vi "Setup measurement.vi"(8 "error in (no error)":errorcluster, 11 "VISA resource name":refnum<visa-resource-name>) -> (0 "error out":errorcluster, 3 "VISA resource name out":refnum<visa-resource-name>)   [LabVIEW 2021]
uses:
  <instrlib>/Keithley 2450/Keithley 2450.lvlib
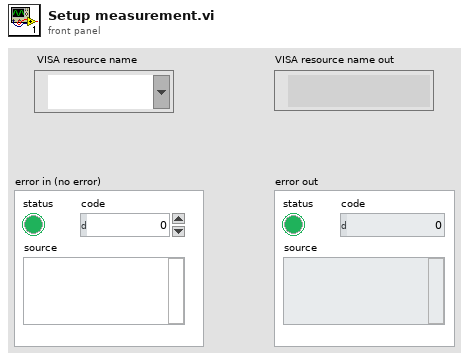
[diagram p1: front panel]
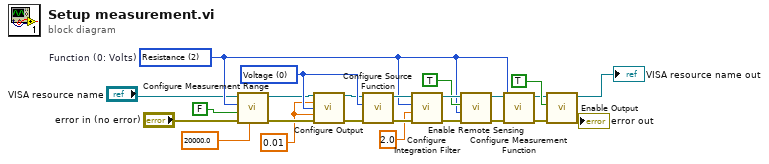
[diagram p0: block diagram]
diagram:
  w24 = u16 0 items=["Voltage", "Current"] ("Source Mode  (0: Voltage)")
  w6 = 0.01 ("Output Level (0)")
  w5 = u16 2 items=["Volts", "Current", "Resistance"]  # Function (0: Volts)
  n1 = call <instrlib>:"Configure Measurement Range.vi"("Manual Range (1.0)"=20000.0 ("Measurement Speed (1 PLC)"), "error in (no error)"="error in (no error)", "Enable Auto Range (T:Enable)"=FALSE, "Function (0: Volts)"=w5, "VISA resource name"="VISA resource name") -> ("error out"=w19:errorcluster, "VISA resource name out"=w20:refnum<visa-resource-name>)  [unwired: 5 in]
  n2 = call <instrlib>:"Configure Output.vi"("VISA resource name"=w20, "Source Level (0)"=w6, "Source Mode  (0: Voltage)"=w24, "Source Limit Level (0.1)"=w6, "error in (no error)"=w19) -> ("VISA resource name out"=w22:refnum<visa-resource-name>, "error out"=w23:errorcluster)  [unwired: 9 in]
  n3 = call <instrlib>:"Configure Source Function.vi"("error in (no error)"=w23, "Function (0: Volts)"=w24, "VISA resource name"=w22) -> ("error out"=w15:errorcluster, "VISA resource name out"=w14:refnum<visa-resource-name>)  [unwired: 7 in]
  n4 = call <instrlib>:"Configure Integration Filter.vi"("error in (no error)"=w15, "Measurement Speed (1 PLC)"=2.0, "Function (0: Volts)"=w5, "VISA resource name"=w14) -> ("error out"=w9:errorcluster, "VISA resource name out"=w10:refnum<visa-resource-name>)  [unwired: 6 in]
  n5 = call <instrlib>:"Enable Remote Sensing.vi"("error in (no error)"=w9, "Function (0:Voltage)"=w5, "Enable Remote Sensing (T: Enable)"=TRUE, "VISA resource name"=w10) -> ("error out"=w12:errorcluster, "VISA resource name out"=w11:refnum<visa-resource-name>)  [unwired: 6 in]
  n6 = call <instrlib>:"Configure Measurement Function.vi"("error in (no error)"=w12, "Function (0: Volts)"=w5, "VISA resource name"=w11) -> ("error out"=w16:errorcluster, "VISA resource name out"=w17:refnum<visa-resource-name>)  [unwired: 7 in]
  n7 = call <instrlib>:"Enable Output.vi"("error in (no error)"=w16, "Enable Output (T: Enable)"=TRUE, "VISA resource name"=w17) -> ("error out"=→"error out":errorcluster, "VISA resource name out"=→"VISA resource name out":refnum<visa-resource-name>)  [unwired: 7 in]
